vi "Convert image array to image.vi"(7 "Error In":errorcluster, 9 "Array":u16[][](array[numeric])) -> (0 "error out":errorcluster, 3 "Image Out":T1)   [LabVIEW 2017]
uses:
  <vilib>/vision/Image Controls.llb/IMAQ Image.ctl
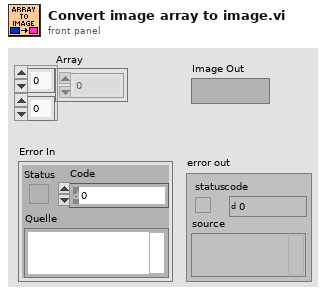
[diagram p1: front panel]
types:
  T1 = typedef "IMAQ Image.ctl" = refnum<image>
  T2 = typedef "Image Type" = u32
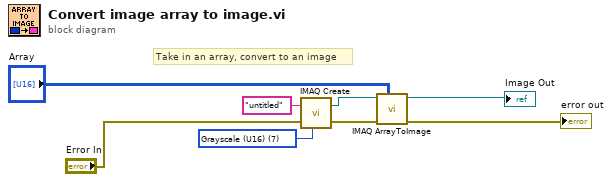
[diagram p0: block diagram]
diagram:
  w8 = T2 7 items=["Grayscale (U8)", "Grayscale (I16)", "Grayscale (SGL)", "Complex (CSG)", "RGB (U32)", "HSL (U32)", "RGB (U64)", "Grayscale (U16)"] ("Image Type")
  # "Take in an array, convert to an image"
  n1 = call "IMAQ Create"("Image Name"="untitled", "Image Type"=w8, "error in (no error)"="Error In") -> ("New Image"=w6:T1, "error out"=w4:errorcluster)  [unwired: 2 in]
  n2 = call "IMAQ ArrayToImage"("Image Pixels (U16)"="Array", "error in (no error)"=w4, "Image"=w6) -> ("error out"=→"error out":errorcluster, "Image Out"=→"Image Out":T1)  [unwired: 7 in]
